vi "encoderfilter.vi"(8 "Encoder Input 4":dbl, 9 "Encoder Input 3":dbl, 10 "Encoder Input 2":dbl, 11 "Encoder Input":dbl) -> (0 "Encoder Output 4":dbl, 1 "Encoder Output 3":dbl, 2 "Encoder Output 2":dbl, 3 "Encoder Output":dbl)   [LabVIEW 2010, in "LASA Beta.lvrbt"]
doc: "Removes bad data from incoder inputs (by replacing any zeros with the last non-zero number)."
uses:
  LASA Beta.lvrbt
panel:
  in  "Last Value 4":dbl
  in  "Last Value 3":dbl
  in  "Last Value 2":dbl
  in  "Last Value":dbl
  # "Last non-zero value of encoders."
  # "ZERO AND MOVING, NOT EXCPECTED"
  # "ZERO AND NOT MOVING, OUTPUT SAME VALUE"
  # "MOVING AND ZERO, OUTPUT LAST NON-ZERO VALUE"
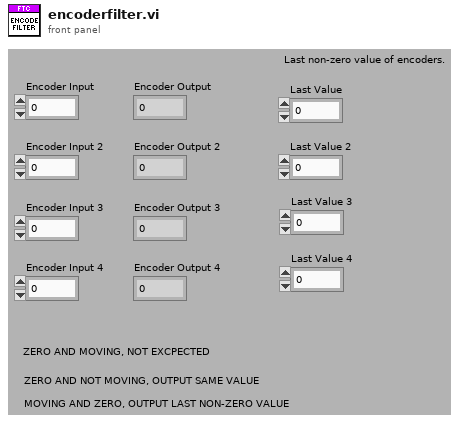
[diagram p1: front panel]
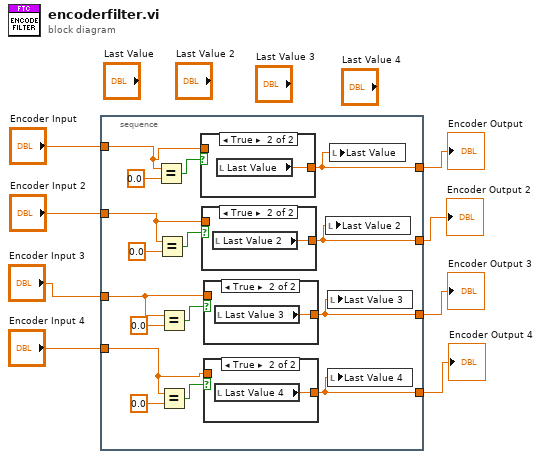
[diagram p0: block diagram]
diagram:
  n1 = stacked-sequence {
    tunnel: "Encoder Input" -> [w21]
    tunnel: [w22] -> w7
    tunnel: "Encoder Input 2" -> [w18]
    tunnel: [w17] -> w5
    tunnel: "Encoder Input 3" -> [w14]
    tunnel: [w13] -> w3
    tunnel: "Encoder Input 4" -> [w10]
    tunnel: [w9] -> w1
    frame #0 {
      n2 = Equal?(x=w21, y=0.0) -> (x = y?=w23:bool)
      n3 = Equal?(x=w18, y=0.0) -> (x = y?=w20:bool)
      n4 = Equal?(x=w14, y=0.0) -> (x = y?=w16:bool)
      n5 = Equal?(x=w10, y=0.0) -> (x = y?=w12:bool)
      n6 = case shown="True" w23 {
        tunnel: [w31 w32] -> w22
        tunnel: w21 -> [w31 _]
        frame False {
        }
        frame True {
          n7 = local read "Last Value"() -> (w32:dbl)
        }
      }
      n8 = case shown="True" w20 {
        tunnel: [w29 w30] -> w17
        tunnel: w18 -> [w29 _]
        frame False {
        }
        frame True {
          n9 = local read "Last Value 2"() -> (w30:dbl)
        }
      }
      n10 = case shown="True" w16 {
        tunnel: [w27 w28] -> w13
        tunnel: w14 -> [w27 _]
        frame False {
        }
        frame True {
          n11 = local read "Last Value 3"() -> (w28:dbl)
        }
      }
      n12 = case shown="True" w12 {
        tunnel: [w25 w26] -> w9
        tunnel: w10 -> [w25 _]
        frame False {
        }
        frame True {
          n13 = local read "Last Value 4"() -> (w26:dbl)
        }
      }
      n14 = local write "Last Value 2"(w17) -> ()
      n15 = local write "Last Value 3"(w13) -> ()
      n16 = local write "Last Value 4"(w9) -> ()
      n17 = local write "Last Value"(w22) -> ()
    }
  }
  "Encoder Output" <- w7
  "Encoder Output 4" <- w1
  "Encoder Output 2" <- w5
  "Encoder Output 3" <- w3
